vi "Find MHL Frames.vi"(8 "error in":errorcluster, 10 "Event Name":string, 11 "References":refnum<vi>[](array[refnum])) -> (0 "error out":errorcluster)   [LabVIEW 2019, in "Panther Dashboard.lvlib"]
uses:
  Panther Dashboard.lvlib
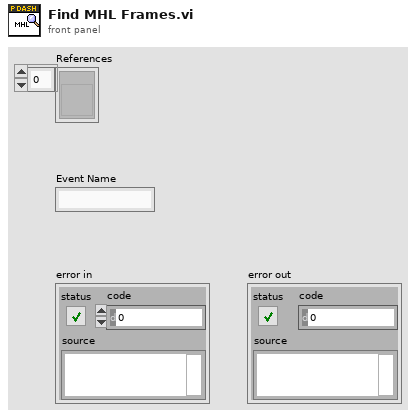
[diagram p1: front panel]
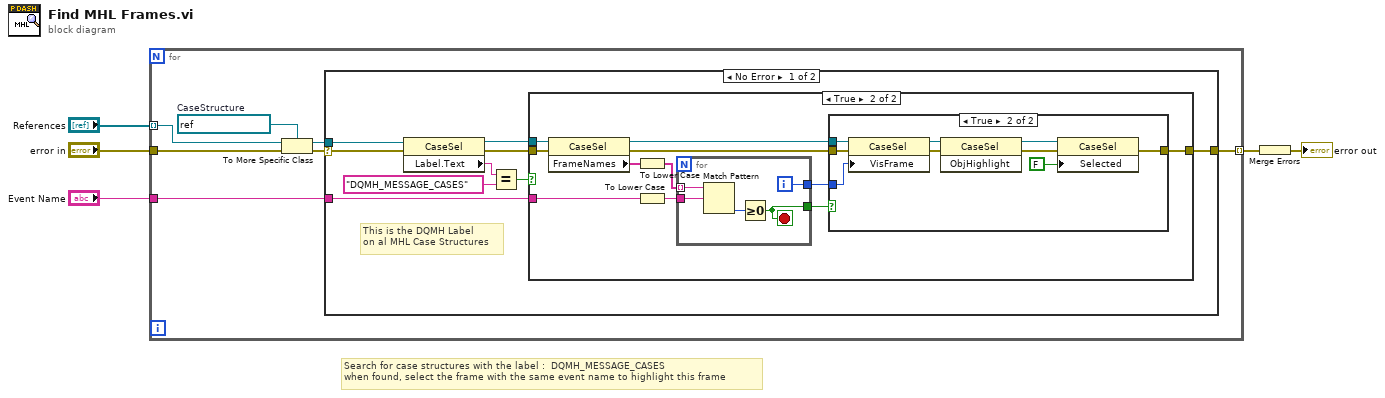
[diagram p0: block diagram]
diagram:
  # "Search for case structures with the label :  DQMH_MESSAGE_CASES\nwhen found, select the frame with the same event name to highlight this frame"
  n1 = for {
    tunnel: "References" -> [w9] mode=indexing
    tunnel: [w11] -> w1 mode=indexing
    tunnel: "Event Name" -> [w6]
    tunnel: "error in" -> [w10]
    w8 = refnum<vi> refnum  # CaseStructure
    n2 = To More Specific Class(target class=w8, reference=w9, error in=w10) -> (specific class reference=w7:refnum<vi>, error out=w12:errorcluster)
    n3 = case shown="No Error" w12 {
      selector: w12 -> [w20 _]
      tunnel: w7 -> [w18 _]
      tunnel: [w21 _] -> w11
      tunnel: w6 -> [w14 _]
      frame No Error {
        # "This is the DQMH Label\non al MHL Case Structures"
        n4 = property class="CaseSel"(reference=w18, error in=w20) -> (reference out=w15:refnum<vi>, error out=w19:errorcluster, "Label.Text"=w13:string)
        n5 = Equal?(x=w13, y="DQMH_MESSAGE_CASES") -> (x = y?=w16:bool)
        n6 = case shown="True" w16 {
          tunnel: [w22 w33] -> w21
          tunnel: w15 -> [_ w30]
          tunnel: w14 -> [_ w25]
          tunnel: w19 -> [w22 w32]
          frame False {
          }
          frame True {
            n7 = property class="CaseSel"(reference=w30, error in=w32) -> (reference out=w27:refnum<vi>, error out=w31:errorcluster, "FrameNames"=w29:string[])
            n8 = To Lower Case(string=w29) -> (all lower case string=w23:string[])
            n9 = To Lower Case(string=w25) -> (all lower case string=w24:string)
            n10 = for {
              tunnel: w23 -> [w44] mode=indexing
              tunnel: w24 -> [w47]
              tunnel: [w48] -> w28
              tunnel: [w45] -> w26
              i -> [w48]
              stop <- w45 stop-if-true
              n11 = Match Pattern(string=w44, regular expression=w47) -> (offset past match=w46:i32)  [unwired: 1 in, 3 out]
              n12 = Greater Or Equal To 0?(x=w46) -> (x >= 0?=w45:bool)
            }
            n13 = case shown="True" w26 {
              tunnel: [w34 w37] -> w33
              tunnel: w31 -> [w34 w41]
              tunnel: w28 -> [_ w39]
              tunnel: w27 -> [_ w38]
              frame False {
              }
              frame True {
                n14 = property class="CaseSel"(reference=w38, error in=w41, "VisFrame"=w39) -> (reference out=w40:refnum<vi>, error out=w43:errorcluster)
                n15 = invoke class="CaseSel" method="ObjHighlight"(reference=w40, error in=w43) -> (reference out=w36:refnum<vi>, error out=w42:errorcluster)  [unwired: 1 in, 1 out]
                n16 = property class="CaseSel"(reference=w36, error in=w42, "Selected"=FALSE) -> (error out=w37:errorcluster)  [unwired: 1 out]
              }
            }
          }
        }
      }
      frame Error {
      }
    }
  }
  n17 = Merge Errors(w1) -> (→"error out":errorcluster)
